vi "Power Spectrum Fractional FFT.vi"(2 "alpha":cdb format="%.2f", 3 "X":cdb[](array[numeric]) format="%.2f") -> (0 "error":i32, 1 "Power Spectrum FFFT {X}":dbl[](array[numeric]) format="%.2f")   [LabVIEW 2017, in "NI_Gmath.lvlib"]
doc: "Realizes the squared magnitude of the fractional fast Fourier transform of complex signals with arbitrarily chosen signal lengths.\n\nIt is\n\nPower Spectrum FFFT = |FFFT{X}(j)|^2 = |Sum exp(-2*pi*i*j*k*alpha)*xk|^2\n\nwhere j and k run from 0 to length(X)."
uses:
  NI_Gmath.lvlib
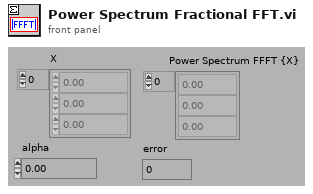
[diagram p1: front panel]
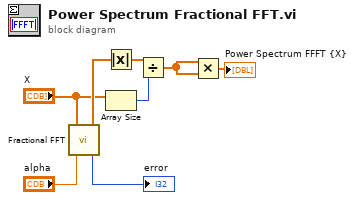
[diagram p0: block diagram]
diagram:
  n1 = call "Fractional FFT.vi"("alpha"="alpha", "X"="X") -> ("error"=→"error":i32, "Fract FFT {X}"=w7:cdb[])
  n2 = Absolute Value(x=w7) -> (abs(x)=w4:dbl[])
  n3 = Array Size(array="X") -> (size(s)=w2:i32)
  n4 = Divide(x=w4, y=w2) -> (x/y=w1:dbl[])
  n5 = Multiply(x=w1, y=w1) -> (x*y=→"Power Spectrum FFFT {X}":dbl[])
